vi "Configure Modulation (Phase).vi"(0 "VISA resource name":refnum<visa-resource-name>, 1 "PM Source (0: Internal)":i32(ring) items=["Internal", "External", "CH1", "CH2"], 2 "Modulation Function (0: Sine)":i32(ring) items=["Sine", "Square", "Ramp", "NRamp", "Triangle", "Noise", "PRBS", "Arbitrary"], 5 "Channel (1: 1)":i32(ring)=1 items=["1"=1, "2"=2], 7 "Enable Phase Modulation(T: Enable)":bool=TRUE, 11 "error in (no error)":errorcluster, 12 "Deviation Degree (180 Degree)":dbl=180.0, 13 "Internal Frequency (10 Hz)":dbl=10.0, 14 "Sample Rate (40000 Sa/s)":dbl=40000.0) -> (4 "VISA resource name out":refnum<visa-resource-name>, 15 "error out":errorcluster)   [LabVIEW 2019, in "Agilent 3352X Series.lvlib"]
doc: "Allows and configures phase modulation. The phase of the carrier is varied by the amplitude of the modulating waveform. The carrier waveform shape and parameters are set by config waveform function.\n\n<b>Note</b>: \n(1) When enabling this mode, all other modes will be turned off.\n(2) The carrier waveform shape and parameters are set by the Configure Standard Waveform VI, Configure PRBS Waveform VI, or Configure Pulse Waveform VI\n(3) You can select a sine, square, ramp, pulse, or PRBS waveform for the carrier (noise, arbitrary waveform, and DC are not allowed)."
uses:
  <instrlib>/Agilent 3352X Series/Agilent 3352X Series.lvlib
panel:
  # "Internal PM Settings"
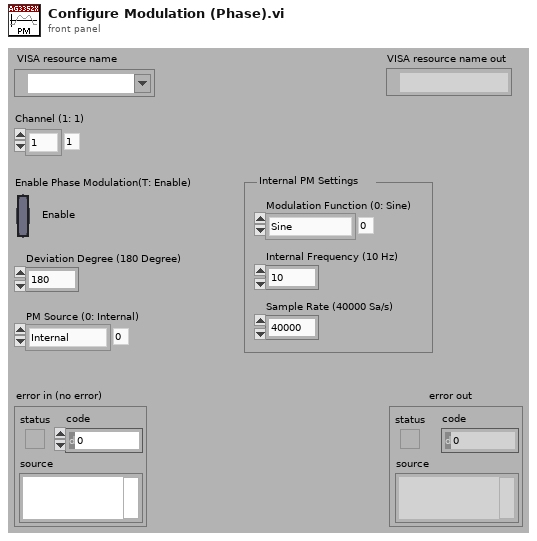
[diagram p1: front panel]
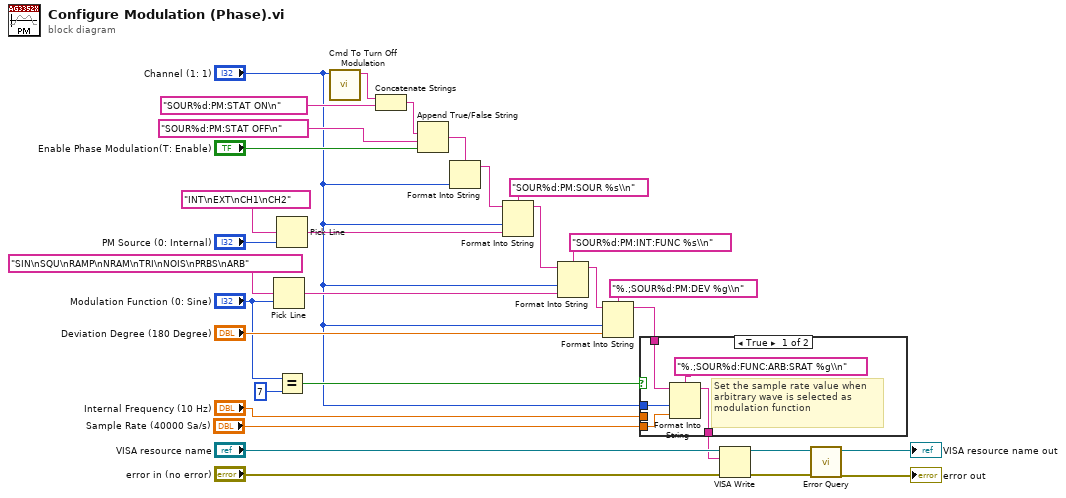
[diagram p0: block diagram]
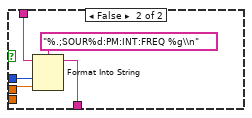
[diagram p2: hidden frame]
diagram:
  n1 = Pick Line(multi-line string="SIN\nSQU\nRAMP\nNRAM\nTRI\nNOIS\nPRBS\nARB", line index="Modulation Function (0: Sine)") -> (output string=w20:string)  [unwired: 1 out]
  n2 = Pick Line(multi-line string="INT\nEXT\nCH1\nCH2", line index="PM Source (0: Internal)") -> (output string=w10:string)  [unwired: 1 out]
  n3 = Equal?(x="Modulation Function (0: Sine)", y=u16 7) -> (x = y?=w13:bool)
  n4 = call <instrlib>:"Cmd To Turn Off Modulation.vi"("Channel (1: 1)"="Channel (1: 1)") -> ("Cmd String"=w6:string)  [unwired: 10 out]
  n5 = Concatenate Strings(w6, "SOUR%d:PM:STAT ON\n") -> (w9:string)
  n6 = Append True/False String(1:"Enable Phase Modulation(T: Enable)", 2:"SOUR%d:PM:STAT OFF\n", 3:w9) -> (0:w8:string)  [unwired: 1 out]
  n7 = Format Into String(format string=w8, "Channel (1: 1)") -> (resulting string=w3:string)  [unwired: 2 in, 1 out]
  n8 = Format Into String(format string="SOUR%d:PM:SOUR %s\\n", initial string=w3, "Channel (1: 1)", w10) -> (resulting string=w17:string)  [unwired: 1 in, 1 out]
  n9 = Format Into String(format string="SOUR%d:PM:INT:FUNC %s\\n", initial string=w17, "Channel (1: 1)", w20) -> (resulting string=w16:string)  [unwired: 1 in, 1 out]
  n10 = Format Into String(format string="%.;SOUR%d:PM:DEV %g\\n", initial string=w16, "Channel (1: 1)", "Deviation Degree (180 Degree)") -> (resulting string=w23:string)  [unwired: 1 in, 1 out]
  n11 = case shown="True" w13 {
    tunnel: "Channel (1: 1)" -> [w35 w42]
    tunnel: w23 -> [w34 w41]
    tunnel: "Internal Frequency (10 Hz)" -> [_ w39]
    tunnel: [w37 w38] -> w21
    tunnel: "Sample Rate (40000 Sa/s)" -> [w33 _]
    frame True {
      # "Set the sample rate value when\narbitrary wave is selected as modulation function"
      n12 = Format Into String(format string="%.;SOUR%d:FUNC:ARB:SRAT %g\\n", initial string=w34, w35, w33) -> (resulting string=w37:string)  [unwired: 1 in, 1 out]
    }
    frame False {
      n13 = Format Into String(format string="%.;SOUR%d:PM:INT:FREQ %g\\n", initial string=w41, w42, w39) -> (resulting string=w38:string)  [unwired: 1 in, 1 out]
    }
  }
  n14 = VISA Write(VISA resource name="VISA resource name", write buffer=w21, error in (no error)="error in (no error)") -> (VISA resource name out=w27:refnum<visa-resource-name>, error out=w26:errorcluster)  [unwired: 1 out]
  n15 = call <instrlib>:"Error Query.vi"("error in (no error)"=w26, "VISA resource name"=w27) -> ("error out"=→"error out":errorcluster, "VISA resource name out"=→"VISA resource name out":refnum<visa-resource-name>)  [unwired: 8 out]
